vi "Sub Process.vi"(8 "error in (no error)":errorcluster, 11 "MPC_AutoInspection in":refnum<class "MPC_AutoInspection.lvclass">) -> (0 "error out":errorcluster, 3 "MPC_AutoInspection out":refnum<class "MPC_AutoInspection.lvclass">)   [LabVIEW 2019, in "MPC_AutoInspection.lvclass"]
uses:
  MPC_AutoInspection.lvclass
  Ctrl/Conveyor Action.ctl
  Ctrl/Station Action.ctl
  FlowCtrl Class/Vision AI/Vision AI.lvclass
  FlowCtrl Class/LineScan/LineScan.lvclass
  MPC_VirbVision/Ctrl/MainPage UI Ref_VirbVision.ctl
  FlowCtrl Class/AI/AI.lvclass
  FlowCtrl Class/BarcodeScan/BarcodeScan.lvclass
  FlowCtrl Class/NG Pick/NG Pick.lvclass
  FlowCtrl Class/Laser Detect/LaserDetect01.lvclass
  Ctrl/Table Save.ctl
  Global/Process Global.vi
  Function/Main UI/Glb/Main_UI Gb.vi
  LLB/Commonly VI/Main Glb.vi
  LLB/Commonly VI.lvlib
panel:
  in  "Boolean 2":bool
  out "Vision AI":T1
  out "error out 2":errorcluster
  out "Boolean":bool
  out "Barcode main":T1
  out "Laser main":T1
  in  "error 2":errorcluster
  out "NG main":T1
  out "AI main":T1
  out "Line main":T1
  in  "NG Pick":T2
  in  "AI":T2
  out "Line Scan":T2
  in  "error":errorcluster
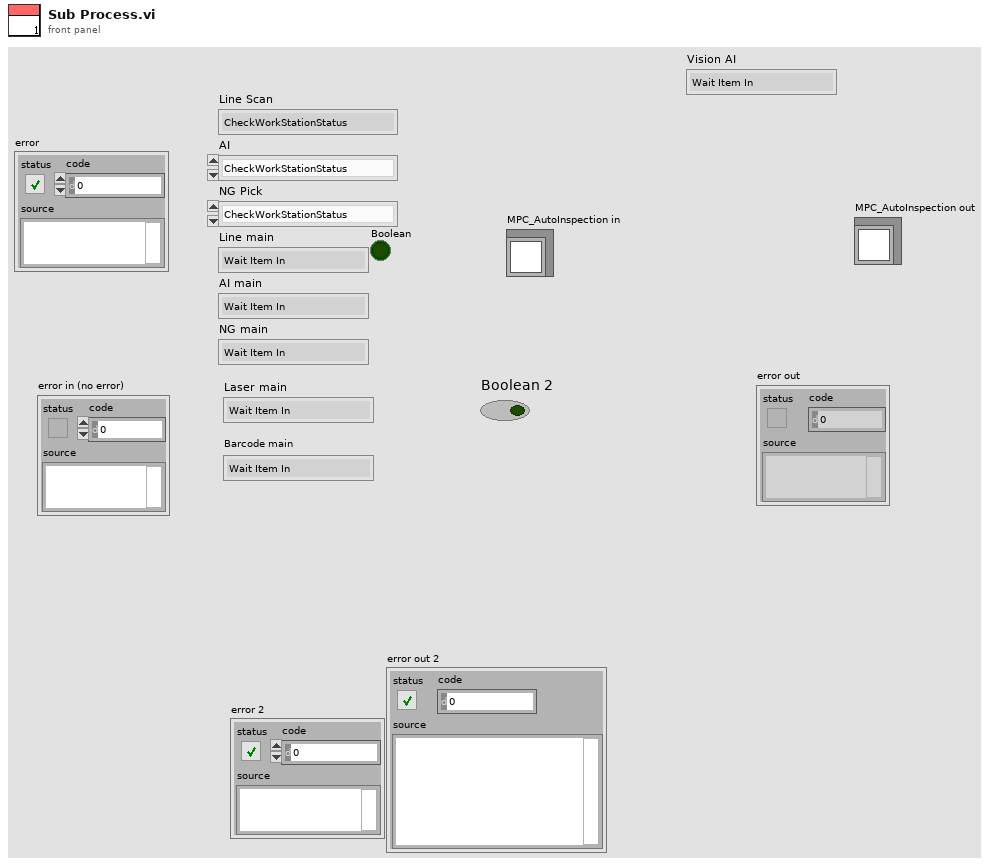
[diagram p1: front panel]
types:
  T1 = typedef "Station Action.ctl" = enum16{"Wait Item In", "Dectect Action", "ImformOut"}
  T2 = typedef "Conveyor Action.ctl" = enum16{"CheckWorkStationStatus", "Request Item In", "Check Product Ready In", "Wait Item In", "Check SlowSignal And Slow", "Check Arrive", "Rise Tray", "FixTray", "Imform Robot", "Wait Robot Imform", "DropTray Imform Out", "Wait Request ", "Flow Out"}
  T3 = typedef "MainPage UI Ref_VirbVision.ctl" = cluster{"ProcessList":refnum<vi>, "Result Arr":refnum<vi>, "StopReceiveCmd":refnum<vi>}
  T4 = enum16{"Chk OK Signal", "Chk NG Signal", "Save OK Log", "Save NG Log", "Del OK Table", "Del NG Table", "Send PLC OK", "Send PLC NG"}
  T5 = typedef "Table Save.ctl" = enum16{"initial", "Add", "Write", "Replace", "Delete", "REad", "RedTable", "Load"}
  T6 = enum16{"Initial", "load", "read", "write", "write sn", "save"}
  T7 = cluster{"ROI":string, "Numbers":i32, "Data":string[][]}[]
  T8 = cluster{"AutoRunFlg":refnum<vi>, "Action Finish Flg":refnum<vi>, "Remaining Action":refnum<vi>, "Btn_AutoRun":refnum<vi>, "Manual Flg":refnum<vi>, "Sub Process Error":refnum<vi>}
  T9 = typedef "SwitchBtn.ctl" = bool
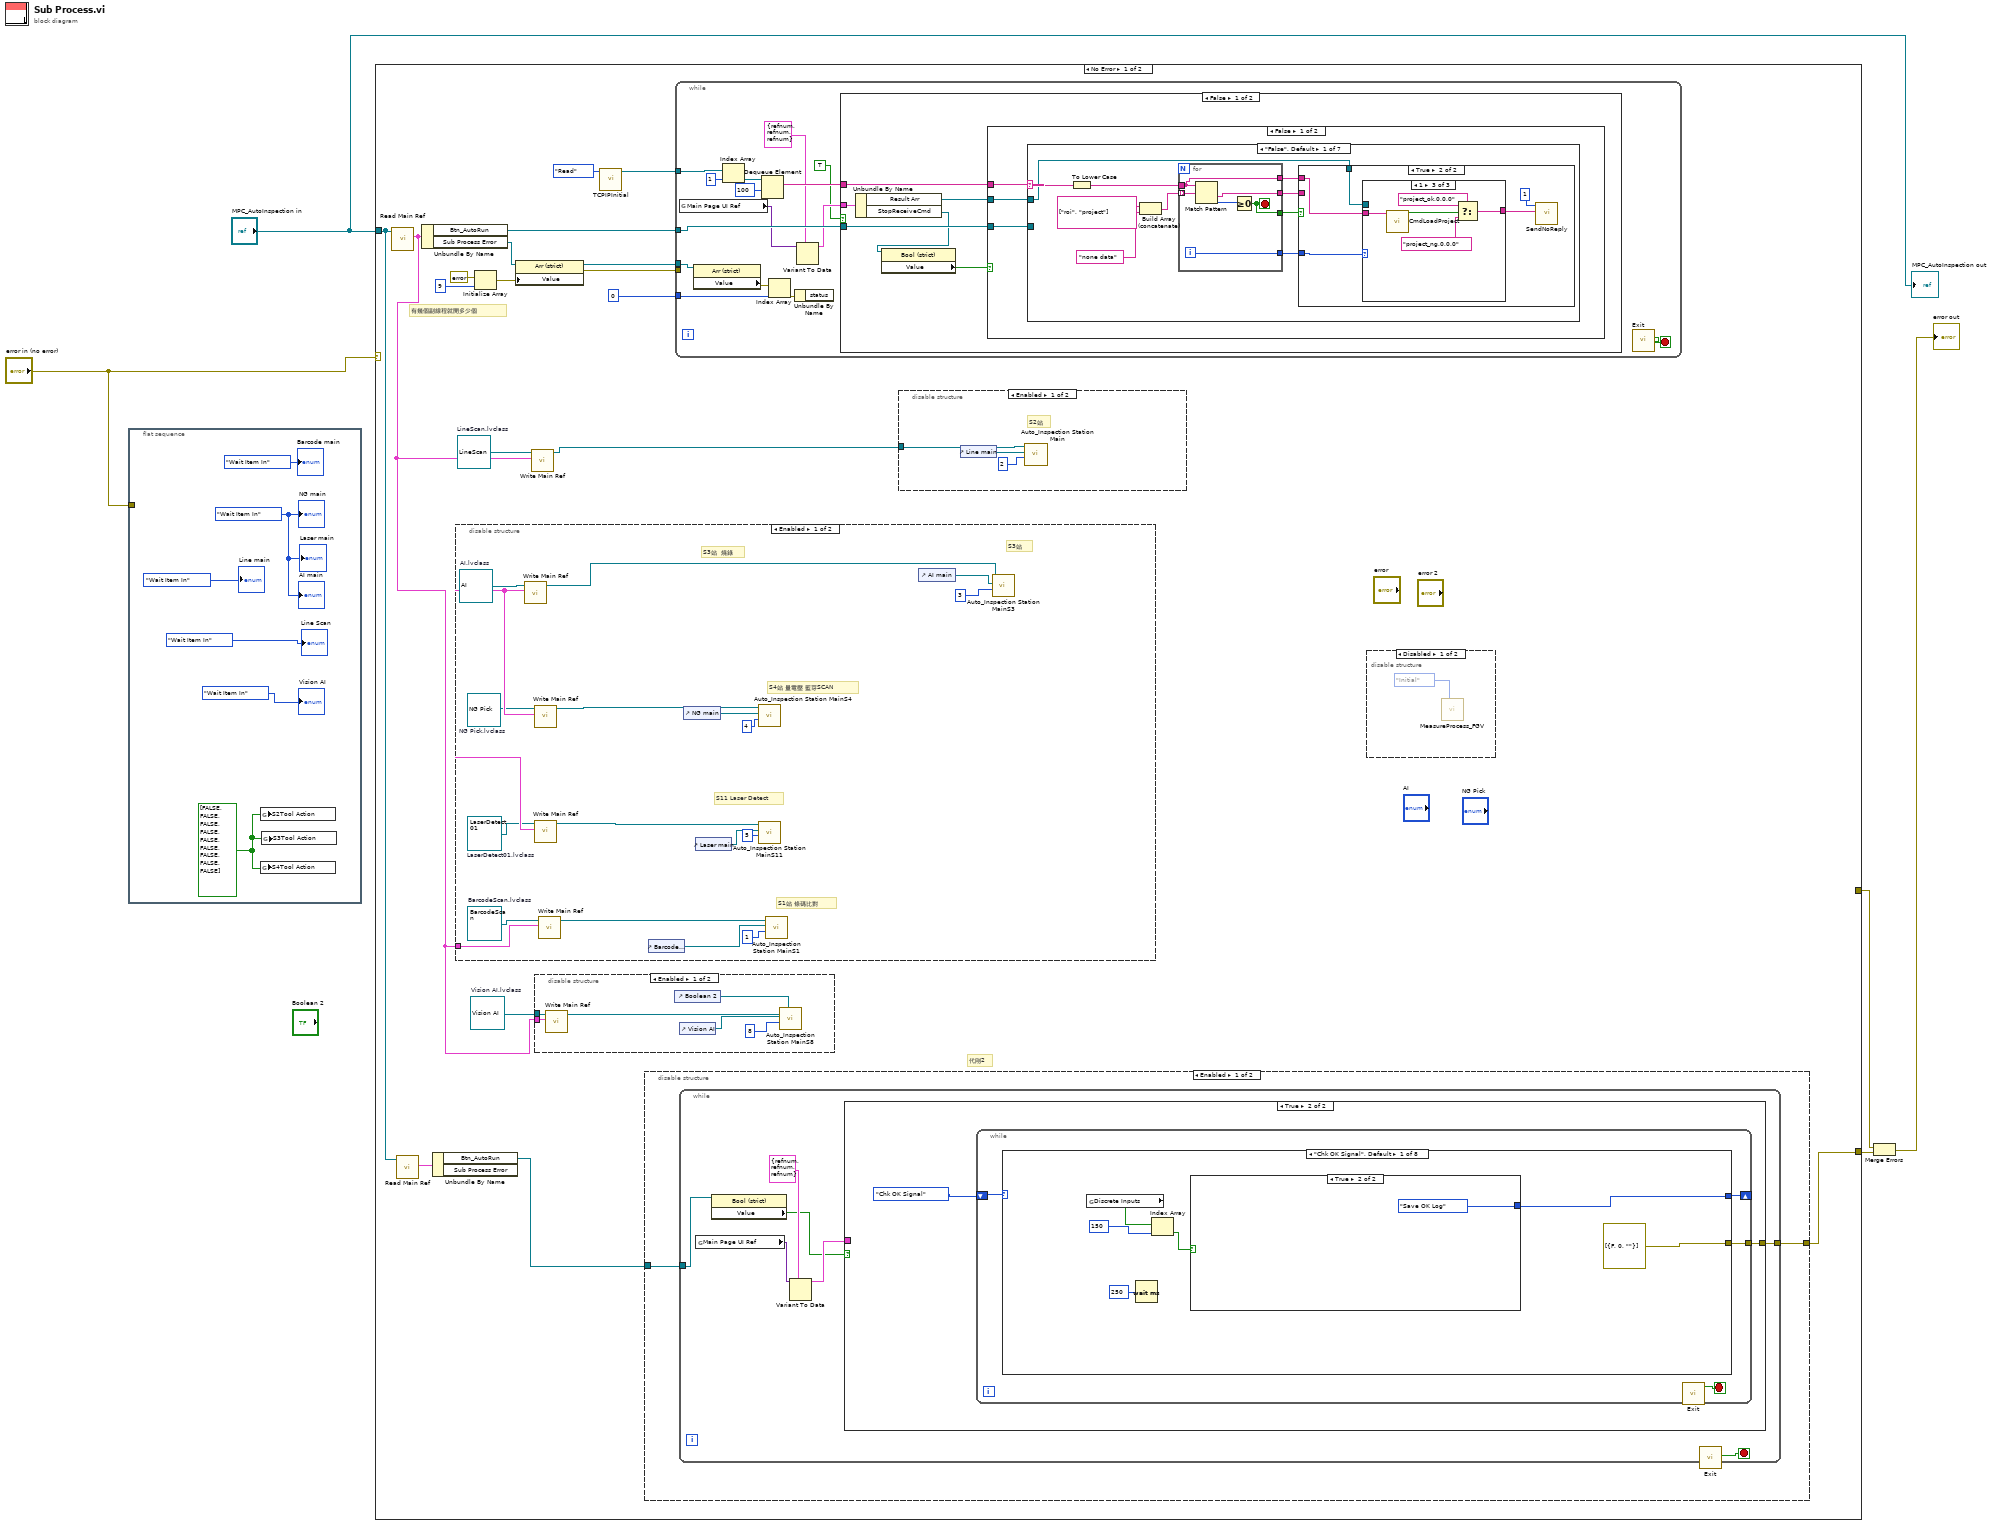
[diagram p0: block diagram]
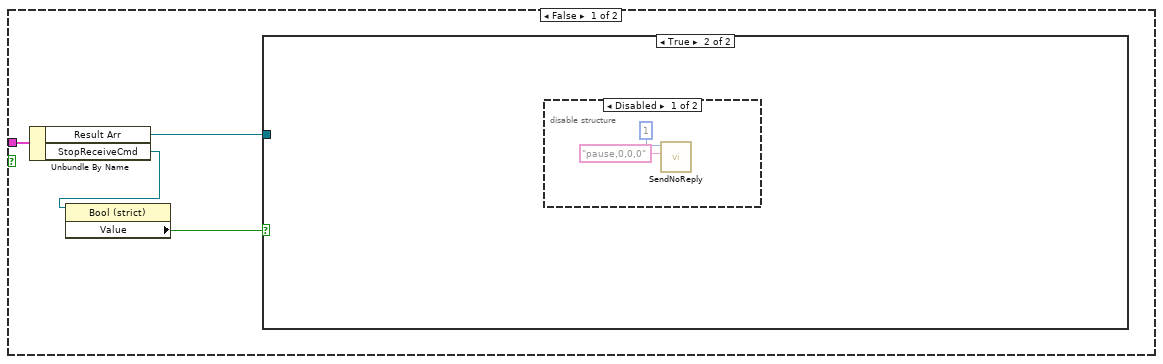
[diagram p2: hidden frame]
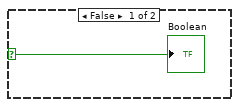
[diagram p3: hidden frame]
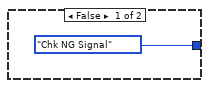
[diagram p5: hidden frame]
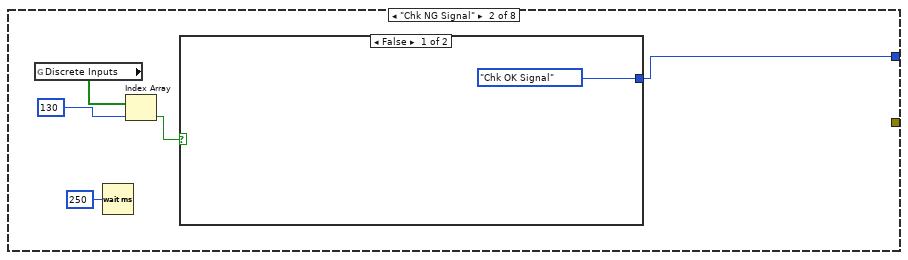
[diagram p6: hidden frame]
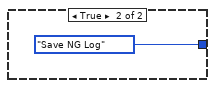
[diagram p7: hidden frame]
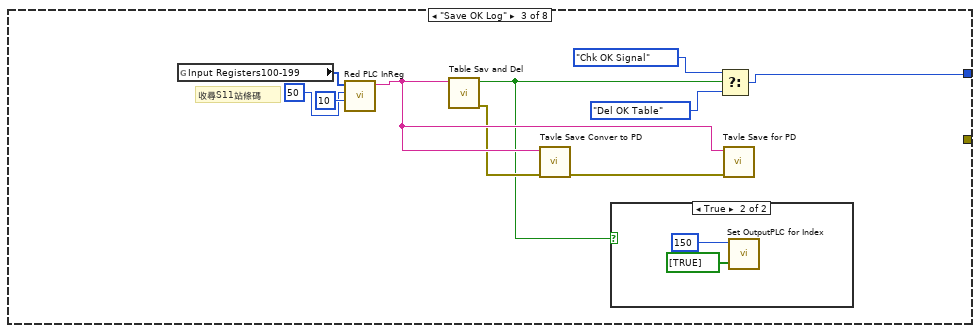
[diagram p8: hidden frame]
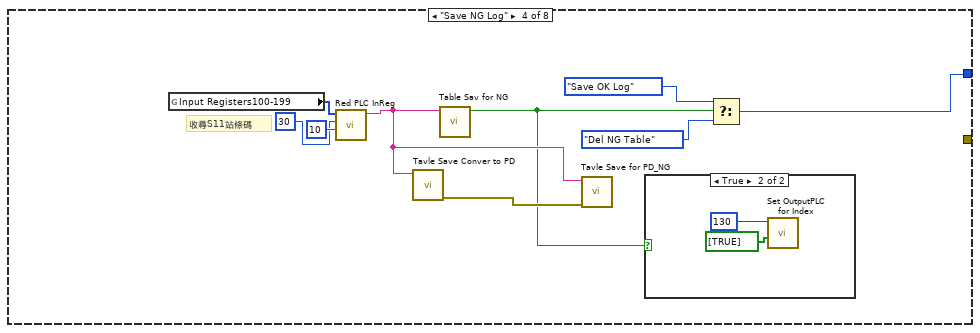
[diagram p10: hidden frame]
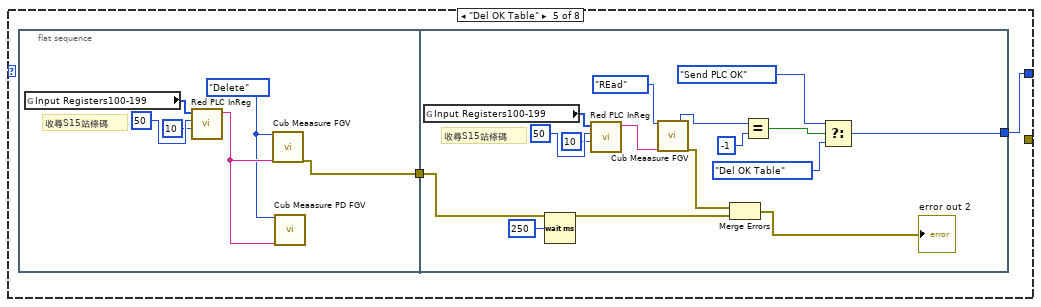
[diagram p12: hidden frame]
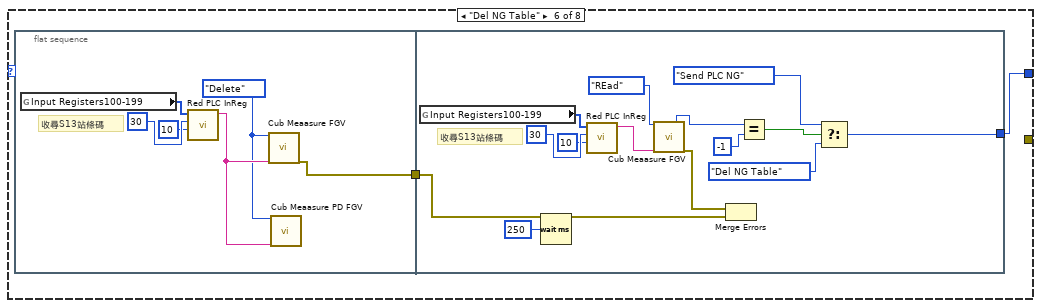
[diagram p13: hidden frame]
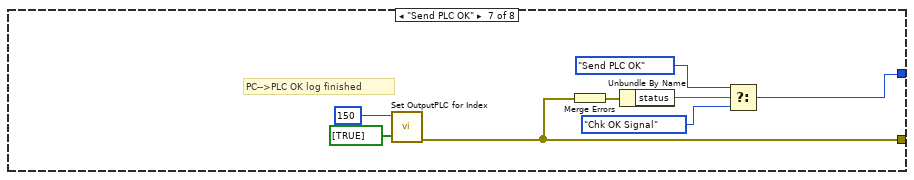
[diagram p14: hidden frame]
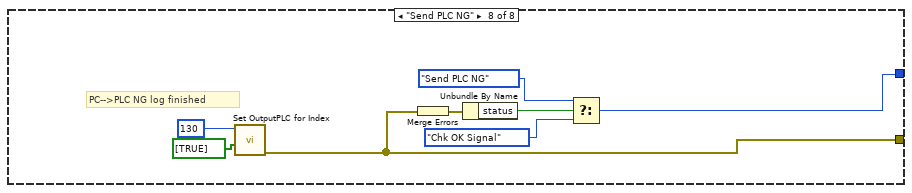
[diagram p15: hidden frame]
diagram:
  n1 = flat-sequence {
    tunnel: "error in (no error)" -> [_]
    frame #0 {
      w7 = bool[] [FALSE, FALSE, FALSE, FALSE, FALSE, FALSE, FALSE, FALSE, FALSE] ("Tool Action")
      w10 = Station_Action."Wait Item In" ("NG main")
      n2 = global write "Process Global.vi" "S2Tool Action"(w7) -> ()
      n3 = global write "Process Global.vi" "S4Tool Action"(w7) -> ()
      n4 = global write "Process Global.vi" "S3Tool Action"(w7) -> ()
      "Barcode main" <- Station_Action."Wait Item In" ("Barcode main")
      "NG main" <- w10
      "Laser main" <- w10
      "AI main" <- w10
      "Line Scan" <- Conveyor_Action."Wait Item In" ("Line Scan")
      "Line main" <- Station_Action."Wait Item In" ("Line main")
      "Vision AI" <- Station_Action."Wait Item In" ("Line main")
    }
  }
  n5 = case shown="No Error" "error in (no error)" {
    selector: "error in (no error)" -> [_ w249]
    tunnel: "MPC_AutoInspection in" -> [w18 _]
    tunnel: [w16 _] -> w3
    tunnel: [_ w249] -> w2
    frame No Error {
      w13 = refnum<class "LineScan.lvclass"> refnum  # LineScan.lvclass
      w15 = refnum<class "Vision AI.lvclass"> refnum  # Vision AI.lvclass
      # "代刚2"
      # "有幾個副線程就開多少個"
      n6 = call-dynamic "Read Main Ref.vi"("Main Process Class in"=w18) -> ("Main Ref"=w14:T8)  [unwired: 8 in, 2 out]
      n7 = call-dynamic "Read Main Ref.vi"("Main Process Class in"=w18) -> ("Main Ref"=w19:T8)  [unwired: 8 in, 2 out]
      n8 = Unbundle By Name(w14) -> ("Btn_AutoRun"=w21:refnum<vi>, "Sub Process Error"=w29:refnum<vi>)
      n9 = Unbundle By Name(w19) -> ("Btn_AutoRun"=w17:refnum<vi>)  [unwired: 1 out]
      n10 = disable-structure shown="Enabled" {
        disable-tunnel: w14 -> [w176 _]
        frame Enabled {
          w167 = refnum<class "LaserDetect01.lvclass"> refnum  # LaserDetect01.lvclass
          w169 = refnum<class "NG Pick.lvclass"> refnum  # NG Pick.lvclass
          w173 = refnum<class "BarcodeScan.lvclass"> refnum  # BarcodeScan.lvclass
          w175 = refnum<class "AI.lvclass"> refnum  # AI.lvclass
          # "S11 Laser Detect"
          # "S4站 量電壓 藍芽SCAN"
          # "S3站"
          # "S1站 條碼比對"
          # "S3站  燒錄"
          n11 = call-dynamic "Write Main Ref.vi"("Main Ref"=w176, "Main Process Class in"=w175) -> ("Main Process Class out"=w174:refnum<class "AI.lvclass">)  [unwired: 8 in, 1 out]
          n12 = call-dynamic "Write Main Ref.vi"("Main Ref"=w176, "Main Process Class in"=w169) -> ("Main Process Class out"=w168:refnum<class "NG Pick.lvclass">)  [unwired: 8 in, 1 out]
          n13 = call-dynamic "Write Main Ref.vi"("Main Ref"=w176, "Main Process Class in"=w167) -> ("Main Process Class out"=w166:refnum<class "LaserDetect01.lvclass">)  [unwired: 8 in, 1 out]
          n14 = call-dynamic "Write Main Ref.vi"("Main Ref"=w176, "Main Process Class in"=w173) -> ("Main Process Class out"=w172:refnum<class "BarcodeScan.lvclass">)  [unwired: 8 in, 1 out]
          n15 = control-ref of="Barcode main"() -> (w171:refnum<vi>)
          n16 = control-ref of="NG main"() -> (w163:refnum<vi>)
          n17 = control-ref of="Laser main"() -> (w161:refnum<vi>)
          n18 = call "Auto_Inspection Station MainS4.vi"("站別"=4, "ActRef"=w163, "Station Action.lvclass"=w168) -> ()  [unwired: 9 in]
          n19 = call "Auto_Inspection Station MainS11.vi"("站別"=5, "ActRef"=w161, "Station Action.lvclass"=w166) -> ()  [unwired: 9 in]
          n20 = call "Auto_Inspection Station MainS1.vi"("站別"=1, "ActRef"=w171, "Station Action.lvclass"=w172) -> ()  [unwired: 9 in]
          n21 = control-ref of="AI main"() -> (w165:refnum<vi>)
          n22 = call "Auto_Inspection Station MainS3.vi"("站別"=3, "ActRef"=w165, "Station Action.lvclass"=w174) -> ()  [unwired: 9 in]
        }
        frame Disabled {
        }
      }
      n23 = Initialize Array(errorcluster {"status"=FALSE, "code"=0, "source"=""} ("error"), 9 ("dimension size")) -> (w27:errorcluster[])
      n24 = property class="Arr (strict)"(reference=w29, "Value"=w27) -> (reference out=w22:refnum<vi>, error out=w20:errorcluster)  [unwired: 1 in]
      n25 = call-dynamic "Write Main Ref.vi"("Main Ref"=w14, "Main Process Class in"=w13) -> ("Main Process Class out"=w12:refnum<class "LineScan.lvclass">)  [unwired: 8 in, 1 out]
      n26 = disable-structure shown="Enabled" {
        disable-tunnel: w15 -> [w156 _]
        disable-tunnel: w14 -> [w155 _]
        frame Enabled {
          n27 = call-dynamic "Write Main Ref.vi"("Main Ref"=w155, "Main Process Class in"=w156) -> ("Main Process Class out"=w153:refnum<class "Vision AI.lvclass">)  [unwired: 8 in, 1 out]
          n28 = control-ref of="Boolean 2"() -> (w151:refnum<vi>)
          n29 = control-ref of="Vision AI"() -> (w154:refnum<vi>)
          n30 = call "Auto_Inspection Station MainS8.vi"("Boolean 2"=w151, "站別"=8, "ActRef"=w154, "Station Action.lvclass"=w153) -> ()  [unwired: 8 in]
        }
        frame Disabled {
        }
      }
      n31 = call "TCPIPInitial.vi"("Enum"=enum16{"initial", "Read", "release"}."Read") -> ("SN_Reply"=w23:refnum<queue>[])  [unwired: 7 in, 3 out]
      n32 = disable-structure shown="Enabled" {
        disable-tunnel: w17 -> [w31 _]
        disable-tunnel: [w30 _] -> w16
        frame Enabled {
          n33 = while {
            tunnel: w31 -> [w34]
            tunnel: [w32] -> w30
            stop <- w38 stop-if-true
            n34 = global read "Main_UI Gb.vi" "Main Page UI Ref"() -> (w35:variant)
            n35 = property class="Bool (strict)"(reference=w34) -> ("Value"=w33:bool)  [unwired: 1 in, 2 out]
            n36 = Variant To Data(type=T3 {"ProcessList"=refnum, "Result Arr"=refnum, "StopReceiveCmd"=refnum} ("Main Page UIRef"), Variant=w35) -> (data=w37:T3)  [unwired: 1 in, 1 out]
            n37 = case shown="True" w33 {
              tunnel: w37 -> [w42 _]
              tunnel: [_ w46] -> w32
              frame False {
                n38 = Unbundle By Name(w42) -> ("Result Arr"=w41:refnum<vi>, "StopReceiveCmd"=w40:refnum<vi>)
                n39 = property class="Bool (strict)"(reference=w40) -> ("Value"=w39:T9)  [unwired: 1 in, 2 out]
                n40 = case shown="True" w39 {
                  selector: w39 -> [w43 _]
                  tunnel: w41 -> [_ _]
                  frame False {
                    "Boolean" <- w43
                  }
                  frame True {
                    n41 = disable-structure shown="Disabled" {
                      frame Disabled {
                        n42 = call "SendNoReply.vi"("DataIn"="pause,0,0,0", "index"=1) -> ()  [unwired: 9 in, 1 out]
                      }
                      frame Enabled {
                      }
                    }
                  }
                }
              }
              frame True {
                n43 = while {
                  shift-right: [w50] -> _
                  shift-left: T4."Chk OK Signal" -> [w49]
                  tunnel: [w48] -> w46
                  stop <- w51 stop-if-true
                  n44 = case shown="\"Chk OK Signal\", Default" w49 {
                    tunnel: [w57 w60 w69 w80 w90 w113 w135 w143] -> w50
                    tunnel: [errorcluster[] [{"status"=FALSE, "code"=0, "source"=""}] ("Error Out") _ _ _ _ _ w140 w144] -> w48
                    frame "Chk OK Signal", Default {
                      n45 = global read "Main Glb.vi" "Discrete Inputs"() -> (w55:bool[])
                      n46 = Wait (ms)(milliseconds to wait=u32 250) -> ()  [unwired: 1 out]
                      n47 = Index Array(array=w55, index=150) -> (element=w53:bool)
                      n48 = case shown="True" w53 {
                        tunnel: [T4."Chk NG Signal" T4."Save OK Log"] -> w57
                        frame False {
                        }
                        frame True {
                        }
                      }
                    }
                    frame "Chk NG Signal" {
                      n49 = global read "Main Glb.vi" "Discrete Inputs"() -> (w63:bool[])
                      n50 = Wait (ms)(milliseconds to wait=u32 250) -> ()  [unwired: 1 out]
                      n51 = Index Array(array=w63, index=130) -> (element=w61:bool)
                      n52 = case shown="False" w61 {
                        tunnel: [T4."Chk OK Signal" T4."Save NG Log"] -> w60
                        frame False {
                        }
                        frame True {
                        }
                      }
                    }
                    frame "Save OK Log" {
                      # "收尋S11站條碼"
                      n53 = global read "Main Glb.vi" "Input Registers100-199"() -> (w76:u16[])
                      n54 = call "Red PLC InReg.vi"("length"=10, "index"=50, "Input Registers Arr"=w76) -> ("Rad In Reg"=w75:string)  [unwired: 7 in, 1 out]
                      n55 = call "Table Sav and Del.vi"("SN"=w75) -> ("error out"=w68:errorcluster, "未找到條碼"=w67:bool)  [unwired: 9 in]
                      n56 = call "Tavle Save Conver to PD .vi"("error in (no error)"=w68, "SN"=w75) -> ("error out 2"=w74:errorcluster)  [unwired: 9 in]
                      n57 = case shown="True" w67 {
                        frame False {
                        }
                        frame True {
                          n58 = call "Set OutputPLC for Index.vi"("Index"=150, "Sat Coils"=bool[] [TRUE]) -> ()  [unwired: 8 in, 1 out]
                        }
                      }
                      n59 = Select(t=T4."Chk OK Signal", s=w67, f=T4."Del OK Table") -> (s? t:f=w69:T4)
                      n60 = call "Tavle Save for PD.vi"("error in (no error)"=w74, "SN"=w75) -> ()  [unwired: 8 in, 2 out]
                    }
                    frame "Save NG Log" {
                      # "收尋S11站條碼"
                      n61 = global read "Main Glb.vi" "Input Registers100-199"() -> (w87:u16[])
                      n62 = call "Red PLC InReg.vi"("length"=10, "index"=30, "Input Registers Arr"=w87) -> ("Rad In Reg"=w86:string)  [unwired: 7 in, 1 out]
                      n63 = call "Tavle Save Conver to PD .vi"("SN"=w86) -> ("error out 2"=w85:errorcluster)  [unwired: 10 in]
                      n64 = call "Table Sav for NG.vi"("SN"=w86) -> ("未找到條碼"=w79:bool)  [unwired: 9 in, 1 out]
                      n65 = call "Tavle Save for PD_NG.vi"("error in (no error)"=w85, "SN"=w86) -> ()  [unwired: 8 in, 2 out]
                      n66 = case shown="True" w79 {
                        frame False {
                        }
                        frame True {
                          n67 = call "Set OutputPLC for Index.vi"("Index"=130, "Sat Coils"=bool[] [TRUE]) -> ()  [unwired: 8 in, 1 out]
                        }
                      }
                      n68 = Select(t=T4."Save OK Log", s=w79, f=T4."Del NG Table") -> (s? t:f=w80:T4)
                    }
                    frame "Del OK Table" {
                      n69 = flat-sequence {
                        tunnel: [w94] -> w91
                        tunnel: [w109] -> w90
                        tunnel: w91 -> [w103]
                        frame #0 {
                          w92 = Table_Save."Delete" ("Action")
                          # "收尋S15站條碼"
                          n70 = global read "Main Glb.vi" "Input Registers100-199"() -> (w95:u16[])
                          n71 = call "Red PLC InReg.vi"("length"=10, "index"=50, "Input Registers Arr"=w95) -> ("Rad In Reg"=w93:string)  [unwired: 7 in, 1 out]
                          n72 = call "Cub Meaasure FGV.vi"("Action"=w92, "SN"=w93) -> ("error out"=w94:errorcluster)  [unwired: 10 in, 7 out]
                          n73 = call "Cub Meaasure PD FGV.vi"("Action"=w92, "SN"=w93) -> ()  [unwired: 10 in, 8 out]
                        }
                        frame #1 {
                          # "收尋S15站條碼"
                          n74 = global read "Main Glb.vi" "Input Registers100-199"() -> (w110:u16[])
                          n75 = Wait (ms)(milliseconds to wait=u32 250) -> ()  [unwired: 1 out]
                          n76 = call "Red PLC InReg.vi"("length"=10, "index"=50, "Input Registers Arr"=w110) -> ("Rad In Reg"=w106:string)  [unwired: 7 in, 1 out]
                          n77 = call "Cub Meaasure FGV.vi"("Action"=Table_Save."REad", "SN"=w106) -> ("條碼的Index"=w104:i32, "error out"=w102:errorcluster)  [unwired: 10 in, 6 out]
                          n78 = Merge Errors(w102, w103) -> (→"error out 2":errorcluster)
                          n79 = Equal?(x=w104, y=-1) -> (x = y?=w101:bool)
                          n80 = Select(t=T4."Send PLC OK", s=w101, f=T4."Del OK Table") -> (s? t:f=w109:T4)
                        }
                      }
                    }
                    frame "Del NG Table" {
                      n81 = flat-sequence {
                        tunnel: [w117] -> w114
                        tunnel: [w131] -> w113
                        tunnel: w114 -> [w125]
                        frame #0 {
                          w115 = Table_Save."Delete" ("Action")
                          # "收尋S13站條碼"
                          n82 = global read "Main Glb.vi" "Input Registers100-199"() -> (w118:u16[])
                          n83 = call "Red PLC InReg.vi"("length"=10, "index"=30, "Input Registers Arr"=w118) -> ("Rad In Reg"=w116:string)  [unwired: 7 in, 1 out]
                          n84 = call "Cub Meaasure FGV.vi"("Action"=w115, "SN"=w116) -> ("error out"=w117:errorcluster)  [unwired: 10 in, 7 out]
                          n85 = call "Cub Meaasure PD FGV.vi"("Action"=w115, "SN"=w116) -> ()  [unwired: 10 in, 8 out]
                        }
                        frame #1 {
                          # "收尋S13站條碼"
                          n86 = global read "Main Glb.vi" "Input Registers100-199"() -> (w132:u16[])
                          n87 = Wait (ms)(milliseconds to wait=u32 250) -> ()  [unwired: 1 out]
                          n88 = call "Red PLC InReg.vi"("length"=10, "index"=30, "Input Registers Arr"=w132) -> ("Rad In Reg"=w128:string)  [unwired: 7 in, 1 out]
                          n89 = call "Cub Meaasure FGV.vi"("Action"=Table_Save."REad", "SN"=w128) -> ("條碼的Index"=w126:i32, "error out"=w124:errorcluster)  [unwired: 10 in, 6 out]
                          n90 = Merge Errors(w124, w125) -> ()  [unwired: 1 out]
                          n91 = Equal?(x=w126, y=-1) -> (x = y?=w123:bool)
                          n92 = Select(t=T4."Send PLC NG", s=w123, f=T4."Del NG Table") -> (s? t:f=w131:T4)
                        }
                      }
                    }
                    frame "Send PLC OK" {
                      # "PC-->PLC OK log finished"
                      n93 = call "Set OutputPLC for Index.vi"("Index"=150, "Sat Coils"=bool[] [TRUE]) -> ("Error Out"=w140:errorcluster[])  [unwired: 8 in]
                      n94 = Merge Errors(w140) -> (w139:errorcluster)
                      n95 = Unbundle By Name(w139) -> ("status"=w138:bool)
                      n96 = Select(t=T4."Send PLC OK", s=w138, f=T4."Chk OK Signal") -> (s? t:f=w135:T4)
                    }
                    frame "Send PLC NG" {
                      # "PC-->PLC NG log finished"
                      n97 = call "Set OutputPLC for Index.vi"("Index"=130, "Sat Coils"=bool[] [TRUE]) -> ("Error Out"=w144:errorcluster[])  [unwired: 8 in]
                      n98 = Merge Errors(w144) -> (w150:errorcluster)
                      n99 = Unbundle By Name(w150) -> ("status"=w149:bool)
                      n100 = Select(t=T4."Send PLC NG", s=w149, f=T4."Chk OK Signal") -> (s? t:f=w143:T4)
                    }
                  }
                  n101 = call "Exit.vi"() -> ("ExitOut"=w51:bool)  [unwired: 11 in]
                }
              }
            }
            n102 = call "Exit.vi"() -> ("ExitOut"=w38:bool)  [unwired: 11 in]
          }
        }
        frame Disabled {
        }
      }
      n103 = while {
        tunnel: w21 -> [w182]
        tunnel: w20 -> [_]
        tunnel: w22 -> [w192]
        tunnel: 0 -> [w190]
        tunnel: w23 -> [w187]
        stop <- w188 stop-if-true
        n104 = global read "Main_UI Gb.vi" "Main Page UI Ref"() -> (w179:variant)
        n105 = property class="Arr (strict)"(reference=w192) -> ("Value"=w191:errorcluster[])  [unwired: 1 in, 2 out]
        n106 = Index Array(array=w187, index=1) -> (element=w185:refnum<queue>)
        n107 = Dequeue Element(queue=w185, timeout in ms (-1)=100) -> (element=w184:string)  [unwired: 1 in, 3 out]
        n108 = Index Array(array=w191, index=w190) -> (element=w189:errorcluster)
        n109 = Unbundle By Name(w189) -> ()  [unwired: 1 out]
        n110 = Variant To Data(type=T3 {"ProcessList"=refnum, "Result Arr"=refnum, "StopReceiveCmd"=refnum} ("Main Page UIRef"), Variant=w179) -> (data=w181:T3)  [unwired: 1 in, 1 out]
        n111 = case shown="False" TRUE {
          tunnel: w184 -> [w198 _]
          tunnel: w182 -> [w197 _]
          tunnel: w181 -> [w196 _]
          frame False {
            n112 = Unbundle By Name(w196) -> ("Result Arr"=w195:refnum<vi>, "StopReceiveCmd"=w194:refnum<vi>)
            n113 = property class="Bool (strict)"(reference=w194) -> ("Value"=w193:T9)  [unwired: 1 in, 2 out]
            n114 = case shown="False" w193 {
              tunnel: w198 -> [w201 _]
              tunnel: w197 -> [w200 _]
              tunnel: w195 -> [w199 _]
              frame False {
                n115 = case shown="\"False\", Default" w201 {
                  selector: w201 -> [w205 _ _ _ _ _ _]
                  tunnel: w200 -> [_ w233 w235 w236 _ _ _]
                  tunnel: w199 -> [w203 _ _ _ w241 w246 _]
                  frame "False", Default {
                    n116 = To Lower Case(string=w205) -> (all lower case string=w204:string)
                    n117 = Build Array (concatenate)(string[] ["roi", "project"], "none data") -> (w209:string[])
                    n118 = for {
                      tunnel: w204 -> [w227]
                      tunnel: w209 -> [w231] mode=indexing
                      tunnel: [w229] -> w206
                      tunnel: [w228] -> w208
                      tunnel: [w227] -> w207
                      tunnel: [w226] -> w202
                      i -> [w229]
                      stop <- w228 stop-if-true
                      n119 = Match Pattern(string=w227, regular expression=w231) -> (after substring=w226:string, offset past match=w230:i32)  [unwired: 1 in, 2 out]
                      n120 = Greater Or Equal To 0?(x=w230) -> (x >= 0?=w228:bool)
                    }
                    n121 = case shown="True" w208 {
                      tunnel: w207 -> [_ w214]
                      tunnel: w206 -> [_ w215]
                      tunnel: w203 -> [_ w216]
                      tunnel: w202 -> [_ _]
                      frame False {
                      }
                      frame True {
                        n122 = case shown="1" w215 {
                          tunnel: w216 -> [_ w220 _]
                          tunnel: w214 -> [_ w219 w225]
                          tunnel: ["" ("SendCmd") w218 w222] -> w213
                          frame Default {
                          }
                          frame 0 {
                            n123 = call "Result To String2.vi"("CmdName"=w219, "Result"=w220) -> ("SendCmd"=w218:string)  [unwired: 9 in]
                          }
                          frame 1 {
                            n124 = call "CmdLoadProject.vi"("String"=w225) -> ("loadok"=w224:bool)  [unwired: 10 in]
                            n125 = Select(t="project_ok,0,0,0", s=w224, f="project_ng,0,0,0") -> (s? t:f=w222:string)
                          }
                        }
                        n126 = call "SendNoReply.vi"("DataIn"=w213, "index"=1) -> ()  [unwired: 9 in, 1 out]
                      }
                    }
                  }
                  frame "Get_OK" {
                    n127 = property class="Bool (strict)"(reference=w233, "Val(Sgnl)"=FALSE ("Value (Signaling)")) -> ()  [unwired: 1 in, 2 out]
                  }
                  frame "trigger" {
                    n128 = property class="Bool (strict)"(reference=w235, "Val(Sgnl)"=TRUE ("Value (Signaling)")) -> ()  [unwired: 1 in, 2 out]
                  }
                  frame "pause" {
                    n129 = flat-sequence {
                      tunnel: w236 -> [w237]
                      frame #0 {
                        n130 = property class="Bool (strict)"(reference=w237, "Val(Sgnl)"=FALSE ("Value (Signaling)")) -> ()  [unwired: 1 in, 2 out]
                      }
                    }
                  }
                  frame "pose" {
                    n131 = call "Result To String.vi"("Result"=w241) -> ("SendCmd"=w239:string)  [unwired: 10 in]
                    n132 = call "SendNoReply.vi"("DataIn"=w239, "index"=1) -> ()  [unwired: 9 in, 1 out]
                  }
                  frame "clear" {
                    n133 = property class="Arr (strict)"(reference=w246, "Value"=T7 []) -> (error out=w243:errorcluster)  [unwired: 1 in, 1 out]
                    n134 = call "SendNoReply.vi"("error in (no error)"=w243, "DataIn"="clear_ok,0,0,0", "index"=1) -> ()  [unwired: 8 in, 1 out]
                  }
                  frame "getall" {
                  }
                }
              }
              frame True {
                n135 = call "SendNoReply.vi"("DataIn"="pause,0,0,0", "index"=1) -> ()  [unwired: 9 in, 1 out]
              }
            }
          }
          frame True {
          }
        }
        n136 = call "Exit.vi"() -> ("ExitOut"=w188:bool)  [unwired: 11 in]
      }
      n137 = disable-structure shown="Enabled" {
        disable-tunnel: w12 -> [w159 _]
        frame Enabled {
          # "S2站"
          n138 = control-ref of="Line main"() -> (w158:refnum<vi>)
          n139 = call "Auto_Inspection Station Main.vi"("站別"=2, "ActRef"=w158, "Station Action.lvclass"=w159) -> ()  [unwired: 9 in]
        }
        frame Disabled {
        }
      }
      n140 = disable-structure shown="Disabled" {
        frame Disabled {
          n141 = call "MeasureProcess_FGV.vi"("action"=T6."Initial") -> ()  [unwired: 10 in, 5 out]
        }
        frame Enabled {
        }
      }
    }
    frame Error {
    }
  }
  n142 = Merge Errors(w2, w3) -> (→"error out":errorcluster)
  "MPC_AutoInspection out" <- "MPC_AutoInspection in"
